vi "Flock_ApplySysConfig_Process.vi"(11 "Process":string="ApplySysConfig") -> ()   [LabVIEW 2014, in "FA_ApplySysConfig.lvlib"]
uses:
  FA_ApplySysConfig.lvlib
  Shared Code/AMC/VI Source/CentralProcessMessaging/Flock_Shared_CentralProcessMessaging.lvlib
  Shared Code/AMC/VI Source/LocalProcessMessaging/Flock_Shared_LocalProcessMessaging.lvlib
  Shared Code/AMC/VI Source/Error Handling/Flock_ErrorHandling.lvlib
panel:
  in  "Stand Alone?":bool
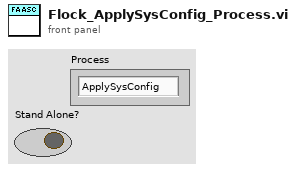
[diagram p1: front panel]
types:
  T1 = typedef "Flock_Shared_Messaging.lvlib/ProcessList.ctl" = string
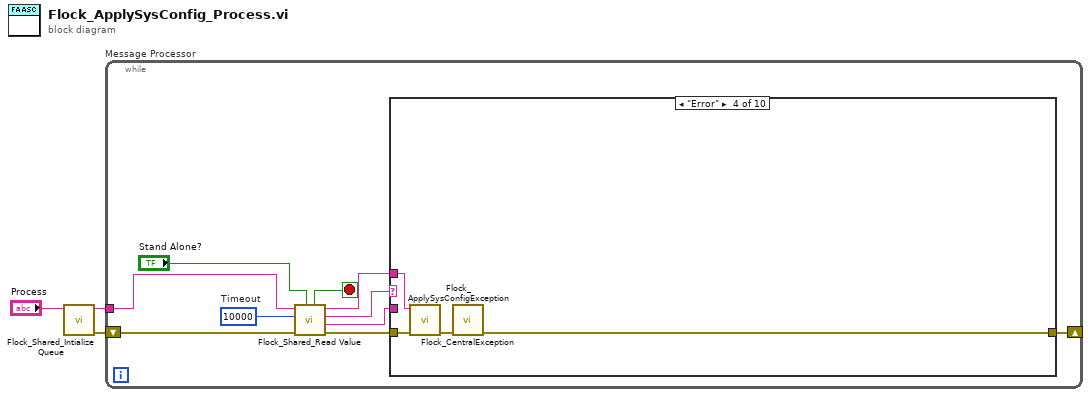
[diagram p0: block diagram]
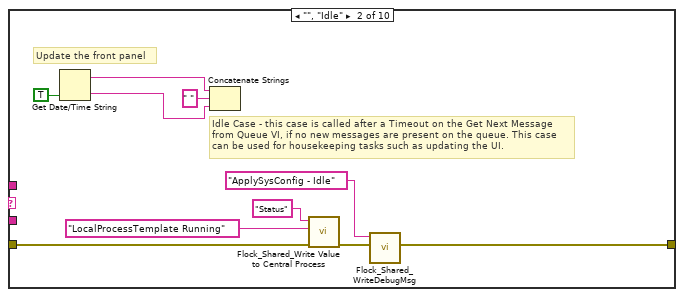
[diagram p3: hidden frame]
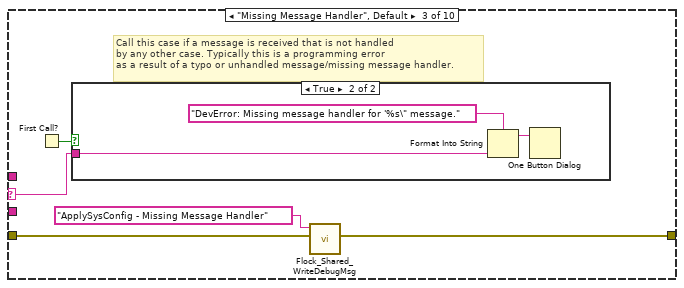
[diagram p4: hidden frame]
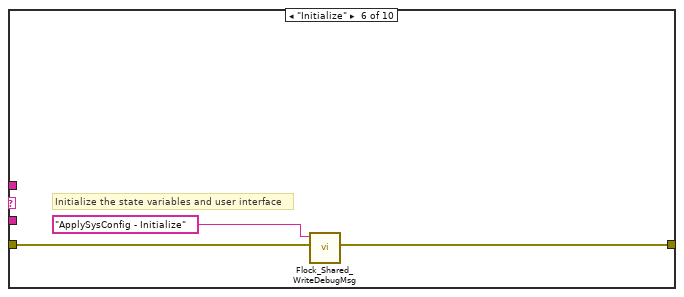
[diagram p7: hidden frame]
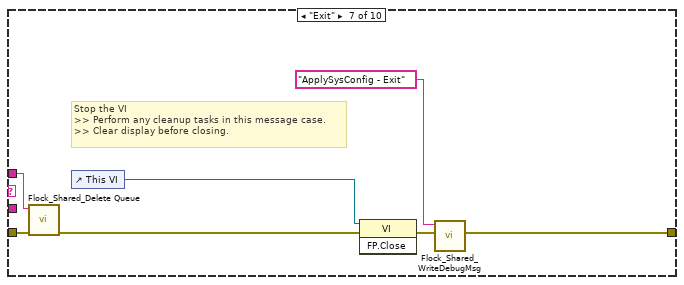
[diagram p8: hidden frame]
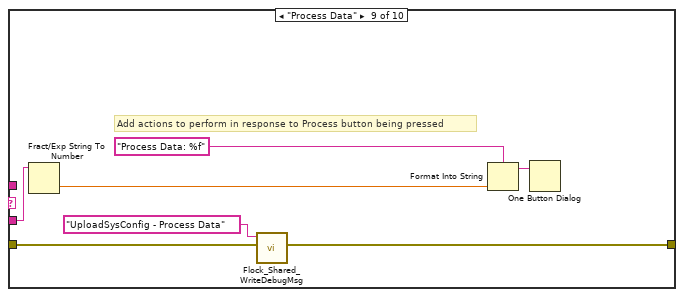
[diagram p10: hidden frame]
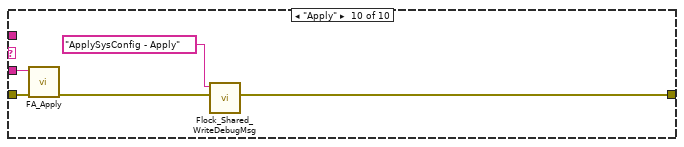
[diagram p11: hidden frame]
diagram:
  n1 = call "Flock_Shared_Intialize Queue.vi"("Enum"="Process") -> ("error out"=w2:errorcluster, "Process Name"=w1:T1)  [unwired: 9 in]
  n2 = while "Message Processor" {
    shift-left: w2 -> [w11]
    shift-right: [w13] -> _
    tunnel: w1 -> [w6]
    stop <- w7 stop-if-true
    w12 = 10000  # Timeout
    n3 = call "Flock_Shared_Read Value.vi"("Stand Alone?"="Stand Alone?", "error in (no error)"=w11, "timeout (1ms)"=w12, "Process"=w6) -> ("error out"=w10:errorcluster, "Message Value"=w8:string, "Message Name"=w9:string, "Process"=w5:T1, "Exit Process"=w7:bool)  [unwired: 3 in]
    n4 = case shown="\"Error\"" w9 {
      selector: w9 -> [_ _ w29 _ _ _ _ _ _ _]
      tunnel: [w14 w16 w27 w36 w37 w40 w43 w48 w50 w59] -> w13
      tunnel: w10 -> [w14 w18 w28 w34 w37 w38 w47 w48 w51 w60]
      tunnel: w8 -> [_ _ _ _ _ _ _ _ w52 w56]
      tunnel: w5 -> [_ _ _ w35 _ _ w46 _ _ _]
      frame "---------- Framework Operations ----------" {
        # "Dummy case to add a seperator in the Case Structure menu"
      }
      frame "", "Idle" {
        # "Update the front panel"
        # "Idle Case - this case is called after a Timeout on the Get Next Message from Queue VI, if no new messages are present on the queue. This case can be used for housekeeping tasks such as updating the UI."
        n5 = Get Date/Time String(want seconds? (F)=TRUE) -> (date string=w24:string, time string=w23:string)  [unwired: 2 out]
        n6 = Concatenate Strings(w24, " " ("string"), w23) -> ()  [unwired: 1 out]
        n7 = call "Flock_Shared_Write Value to Central Process.vi"("error in (no error)"=w18, "Message Value"="LocalProcessTemplate Running", "Message Name"="Status") -> ("error out"=w17:errorcluster)  [unwired: 8 in]
        n8 = call "Flock_Shared_WriteDebugMsg.vi"("error in (no error)"=w17, "Current Message Case"="ApplySysConfig - Idle") -> ("error out"=w16:errorcluster)  [unwired: 9 in]
      }
      frame "Missing Message Handler", Default {
        # "Call this case if a message is received that is not handled \nby any other case. Typically this is a programming error\nas a result of a typo or unhandled message/missing message handler."
        n9 = First Call?() -> (First Call?: T/F=w25:bool)
        n10 = case shown="True" w25 {
          tunnel: w29 -> [_ w32]
          frame False {
          }
          frame True {
            n11 = Format Into String(format string="DevError: Missing message handler for '%s\" message." ("message"), w32) -> (resulting string=w30:string)  [unwired: 2 in, 1 out]
            n12 = One Button Dialog(message=w30) -> ()  [unwired: 2 out]
          }
        }
        n13 = call "Flock_Shared_WriteDebugMsg.vi"("error in (no error)"=w28, "Current Message Case"="ApplySysConfig - Missing Message Handler") -> ("error out"=w27:errorcluster)  [unwired: 9 in]
      }
      frame "Error" {
        n14 = call "Flock_ApplySysConfigException.vi"("Error In"=w34, "Process List"=w35) -> ("Error Out"=w33:errorcluster)  [unwired: 9 in]
        n15 = call "Flock_CentralException.vi"("Error In"=w33) -> ("Error Out"=w36:errorcluster)  [unwired: 10 in]
      }
      frame "---------- Generic Operations ----------" {
        # "Dummy case to add a seperator in the Case Structure menu"
      }
      frame "Initialize" {
        # "Initialize the state variables and user interface"
        n16 = call "Flock_Shared_WriteDebugMsg.vi"("error in (no error)"=w38, "Current Message Case"="ApplySysConfig - Initialize") -> ("error out"=w40:errorcluster)  [unwired: 9 in]
      }
      frame "Exit" {
        # "Stop the VI\n>> Perform any cleanup tasks in this message case.\n>> Clear display before closing."
        n17 = call "Flock_Shared_Delete Queue.vi"("Error In"=w47, "Process Name"=w46) -> ("Error Out"=w44:errorcluster)  [unwired: 9 in]
        n18 = control-ref of="This VI"() -> (w45:refnum<vi>)
        n19 = invoke class="VI" method="FP.Close"(reference=w45, error in=w44) -> (error out=w41:errorcluster)  [unwired: 1 in, 2 out]
        n20 = call "Flock_Shared_WriteDebugMsg.vi"("error in (no error)"=w41, "Current Message Case"="ApplySysConfig - Exit") -> ("error out"=w43:errorcluster)  [unwired: 9 in]
      }
      frame "---------- Application Operations ----------" {
        # "Dummy case to add a seperator in the Case Structure menu"
      }
      frame "Process Data" {
        # "Add actions to perform in response to Process button being pressed"
        n21 = Fract/Exp String To Number(string=w52) -> (number=w55:dbl)  [unwired: 4 out]
        n22 = call "Flock_Shared_WriteDebugMsg.vi"("error in (no error)"=w51, "Current Message Case"="UploadSysConfig - Process Data") -> ("error out"=w50:errorcluster)  [unwired: 9 in]
        n23 = Format Into String(format string="Process Data: %f" ("message"), w55) -> (resulting string=w53:string)  [unwired: 2 in, 1 out]
        n24 = One Button Dialog(message=w53) -> ()  [unwired: 2 out]
      }
      frame "Apply" {
        n25 = call "FA_Apply.vi"("Error In"=w60, "Special Type"=w56) -> ("Error Out"=w57:errorcluster)  [unwired: 9 in]
        n26 = call "Flock_Shared_WriteDebugMsg.vi"("error in (no error)"=w57, "Current Message Case"="ApplySysConfig - Apply") -> ("error out"=w59:errorcluster)  [unwired: 9 in]
      }
    }
  }
